vi "Set OP and Post OP Measurements.vi"(8 "error in (no error)":errorcluster, 11 "Servo MSMT in":refnum<class "Servo MSMT.lvclass">) -> (0 "error out":errorcluster, 3 "Servo MSMT out":refnum<class "Servo MSMT.lvclass">)   [LabVIEW 2018, in "Servo MSMT.lvlib" / "Servo MSMT.lvclass"]
uses:
  Servo MSMT.lvclass
  C:/Sequence Automation/Plugins/Measurement Interface.lvlibp/Measurement Interface.lvclass
  Servo MSMT.lvclass/Servo MSMT.ctl
  Read DC Pins.vi
  Write Servo Measurements.vi
  Plugins/Measurement Interface.lvlibp/Private Methods/Measurement Parameters/Read Measurement Parameters.vi
  Plugins/String Database.lvlibp/String Database.lvclass
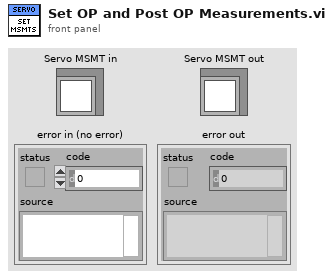
[diagram p1: front panel]
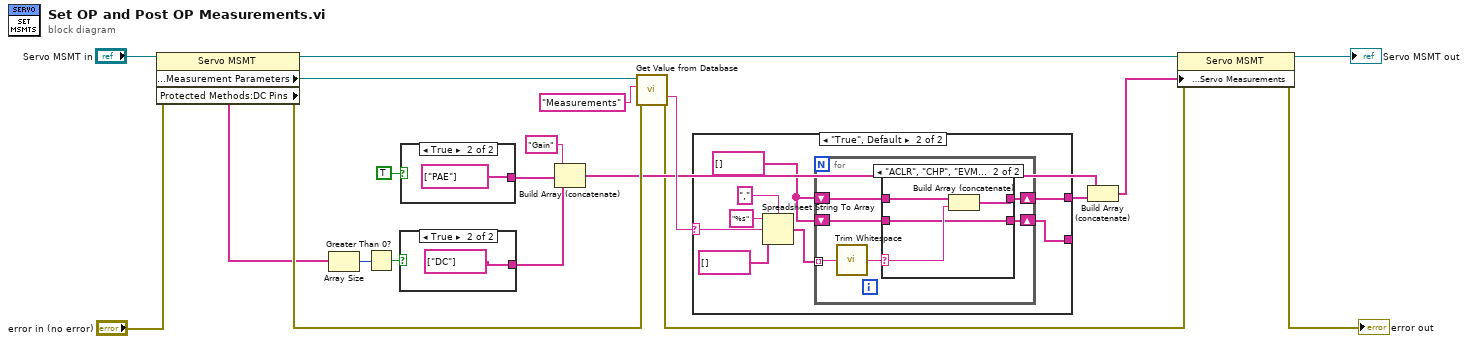
[diagram p0: block diagram]
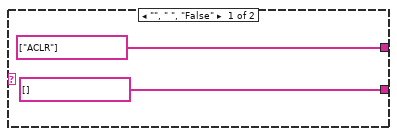
[diagram p2: hidden frame]
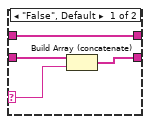
[diagram p3: hidden frame]
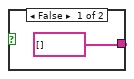
[diagram p4: hidden frame]
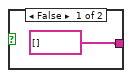
[diagram p5: hidden frame]
diagram:
  n1 = property class="Servo MSMT"(reference="Servo MSMT in", error in="error in (no error)") -> (reference out=w17:refnum<class "Servo MSMT.lvclass">, error out=w18:errorcluster, "Protected Methods:Measurement Parameters"=w20:refnum<class "String Database.lvclass">, "Protected Methods:DC Pins"=w16:string[])
  n2 = Array Size(array=w16) -> (size(s)=w15:i32)
  n3 = Greater Than 0?(x=w15) -> (x > 0?=w14:bool)
  n4 = case shown="True" w14 {
    tunnel: [string[] [] string[] ["DC"]] -> w8
    frame False {
    }
    frame True {
    }
  }
  n5 = case shown="True" TRUE {
    tunnel: [string[] [] string[] ["PAE"]] -> w13
    frame False {
    }
    frame True {
    }
  }
  n6 = Build Array (concatenate)("Gain" ("Entry Name"), w13, w8) -> (w11:string[])
  n7 = call "Get Value from Database.vi"("error in (no error)"=w18, "Entry Name"="Measurements", "Message in"=w20) -> ("error out"=w4:errorcluster, "Entry Value"=w12:string)  [unwired: 5 in, 2 out]
  n8 = case shown="\"True\", Default" w12 {
    selector: w12 -> [_ w33]
    tunnel: [string[] ["ACLR"] w29] -> w10
    tunnel: [string[] [] w27] -> _
    frame "", " ", "False" {
    }
    frame "True", Default {
      w28 = string[] []
      n9 = Spreadsheet String To Array(delimiter (Tab)=",", format string="%s", spreadsheet string=w33, array type (2D Dbl)=string[] []) -> (array=w30:string[])
      n10 = for {
        tunnel: w30 -> [w36] mode=indexing
        shift-right: [w40] -> w29
        shift-left: w28 -> [w39]
        shift-right: [w37] -> w27
        shift-left: w28 -> [w38]
        n11 = call <vilib>:"Trim Whitespace.vi"("string"=w36) -> ("trimmed string"=w35:string)  [unwired: 1 in]
        n12 = case shown="\"ACLR\", \"CHP\", \"EVM\", \"ModAcc\", \"OBW\", \"ORFS\", \"PFER\", \"PVT\", \"SEM\"" w35 {
          selector: w35 -> [w41 w47]
          tunnel: [w44 w46] -> w40
          tunnel: w39 -> [w44 w48]
          tunnel: w38 -> [w43 w45]
          tunnel: [w42 w45] -> w37
          frame "False", Default {
            n13 = Build Array (concatenate)(w43, w41) -> (w42:string[])
          }
          frame "ACLR", "CHP", "EVM", "ModAcc", "OBW", "ORFS", "PFER", "PVT", "SEM" {
            n14 = Build Array (concatenate)(w48, w47) -> (w46:string[])
          }
        }
      }
    }
  }
  n15 = Build Array (concatenate)(w11, w10) -> (w1:string[])
  n16 = property class="Servo MSMT"(reference=w17, error in=w4, "Protected Methods:Servo Measurements"=w1) -> (reference out=→"Servo MSMT out":refnum<class "Servo MSMT.lvclass">, error out=→"error out":errorcluster)
